vi "Run.vi"() -> (0 "error out":errorcluster)   [LabVIEW 2013]
uses:
  ModeType.ctl
  OutputDirectory.vi
panel:
  in  "pattern":string="*.vi"
  out "Running Test Number":i32
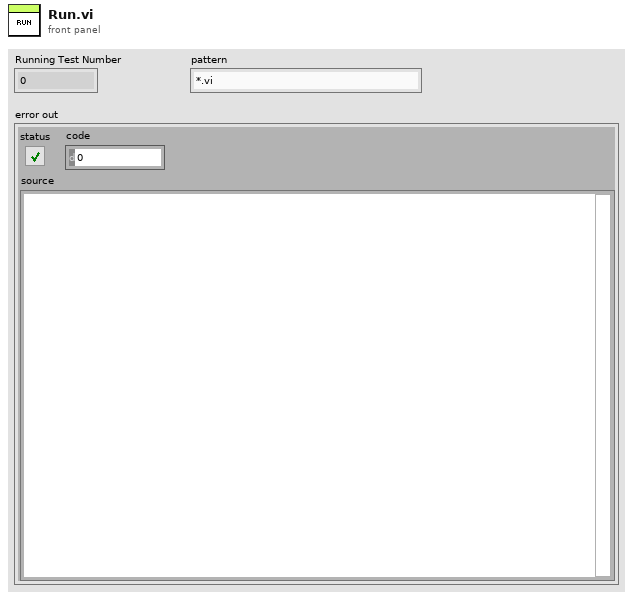
[diagram p1: front panel]
types:
  T1 = typedef "ModeType.ctl" = enum16{"Normal", "Expected Failure", "Skipped", "Broken"}
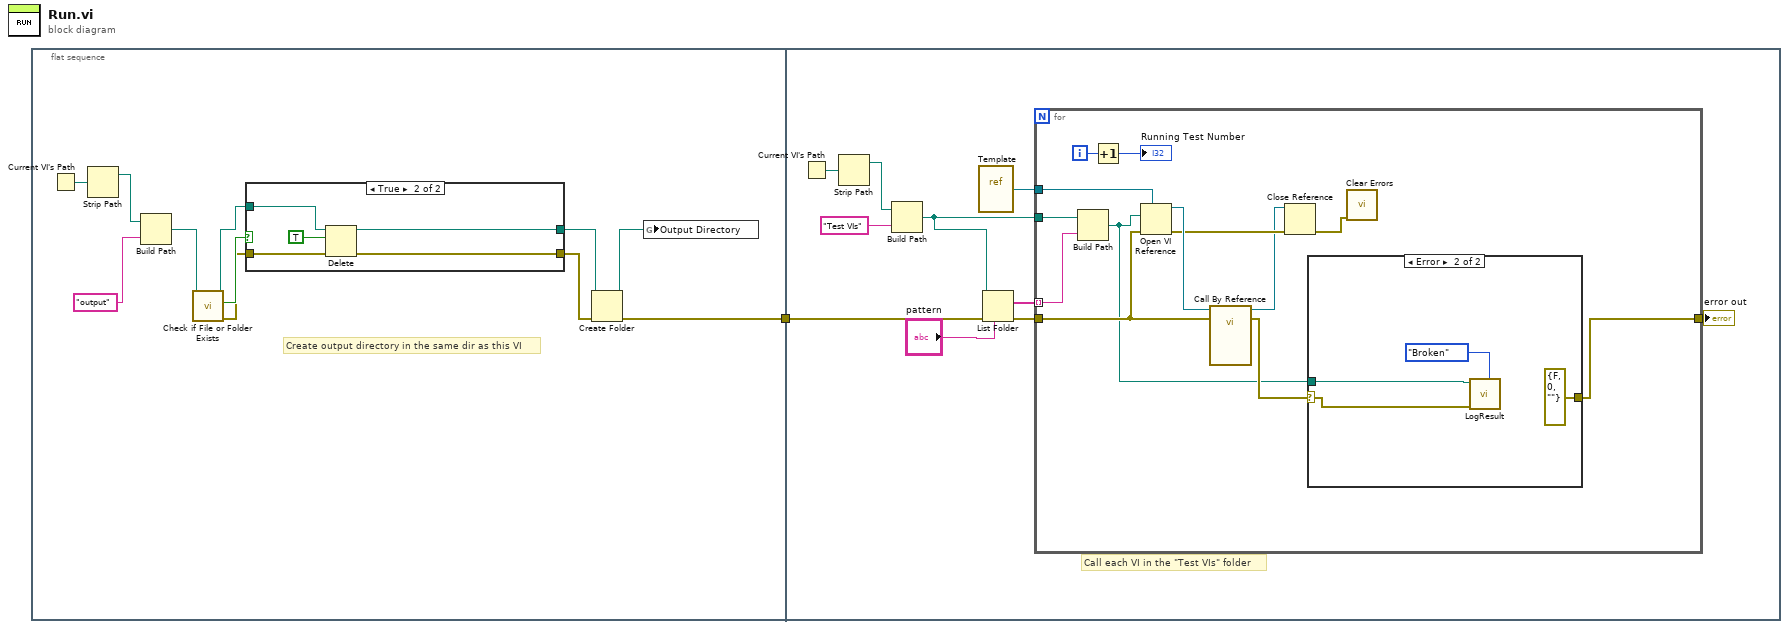
[diagram p0: block diagram]
diagram:
  n1 = flat-sequence {
    tunnel: [w2] -> w1
    tunnel: w1 -> [w21]
    frame #0 {
      # "Create output directory in the same dir as this VI"
      n2 = Current VI's Path() -> (path=w12:path)
      n3 = Strip Path(path=w12) -> (stripped path=w11:path)  [unwired: 1 out]
      n4 = Build Path(base path=w11, name or relative path="output") -> (appended path=w9:path)
      n5 = call <vilib>:"Check if File or Folder Exists.vi"("path"=w9) -> ("error out"=w4:errorcluster, "file or folder exists?"=w8:bool, "dup path"=w7:path)  [unwired: 8 in]
      n6 = case shown="True" w8 {
        tunnel: w7 -> [w14 w19]
        tunnel: [w14 w17] -> w6
        tunnel: w4 -> [w13 w16]
        tunnel: [w13 w15] -> w3
        frame False {
        }
        frame True {
          n7 = Delete(path (use dialog)=w19, entire hierarchy (F)=TRUE, error in=w16) -> (deleted path=w17:path, error out=w15:errorcluster)  [unwired: 2 in, 1 out]
        }
      }
      n8 = Create Folder(path (use dialog)=w6, error in=w3) -> (created path=w5:path, error out=w2:errorcluster)  [unwired: 1 in, 1 out]
      n9 = global write "OutputDirectory.vi" "Output Directory"(w5) -> ()
    }
    frame #1 {
      # "Call each VI in the \"Test VIs\" folder"
      n10 = Current VI's Path() -> (path=w29:path)
      n11 = Strip Path(path=w29) -> (stripped path=w28:path)  [unwired: 1 out]
      n12 = Build Path(base path=w28, name or relative path="Test VIs") -> (appended path=w23:path)
      n13 = vi-ref "Template.vi"() -> (w24:refnum<vi>)
      n14 = List Folder(path=w23, pattern="pattern", error in=w21) -> (filenames=w25:string[], error out=w20:errorcluster)  [unwired: 1 in, 2 out]
      n15 = for {
        tunnel: w25 -> [w40] mode=indexing
        tunnel: w24 -> [w42]
        tunnel: w23 -> [w41]
        tunnel: [w32] -> w22
        tunnel: w20 -> [w34]
        i -> [w36]
        n16 = Build Path(base path=w41, name or relative path=w40) -> (appended path=w31:path)
        n17 = Increment(x=w36) -> (x+1=→"Running Test Number":i32)
        n18 = Open VI Reference(type specifier VI Refnum (for type only)=w42, vi path=w31, error in (no error)=w34) -> (vi reference=w39:refnum<vi>, error out=w38:errorcluster)  [unwired: 3 in]
        n19 = call-by-ref "?"(reference=w39, error in=w34) -> (reference out=w37:refnum<vi>, error out=w33:errorcluster)  [unwired: 12 in]
        n20 = Close Reference(reference=w37, error in (no error)=w38) -> (error out=w30:errorcluster)
        n21 = case shown="Error" w33 {
          selector: w33 -> [w43 w44]
          tunnel: [w43 errorcluster {"status"=FALSE, "code"=0, "source"=""} ("error IO")] -> w32
          tunnel: w31 -> [_ w47]
          frame No Error {
          }
          frame Error {
            n22 = call "LogResult.vi"("Mode"=ModeType."Broken", "Test Result"=w44, "VI Path"=w47) -> ()  [unwired: 9 in]
          }
        }
        n23 = call <vilib>:"Clear Errors.vi"("error in (no error)"=w30) -> ()  [unwired: 6 in, 1 out]
      }
      "error out" <- w22
    }
  }
